vi "Dialog_Arrow Key Handler.vi"(9 "Done Ref":refnum<vi>, 10 "Filter String Ref":refnum<vi>, 11 "Tree Ref":refnum<vi>[](array[refnum])) -> ()   [LabVIEW 2023]
doc: "Called asynchronously, this VI sets the default string (default=\"Filter...\") and the secondary color to the control's text color (default = gray), then monitors the control for a change in focus. When control gains focus, it removes the default string and sets the text to the main text color. When it loses focus, and if string is empty, it sets the value to the default and sets secondary text color.\n\nMake key focus will place the cursor before the default text and handle removing default text if user types any ascii character"
panel:
  in  "Tree":string[](tree)
  in  "Filter String":string
  # "Debug controls:"
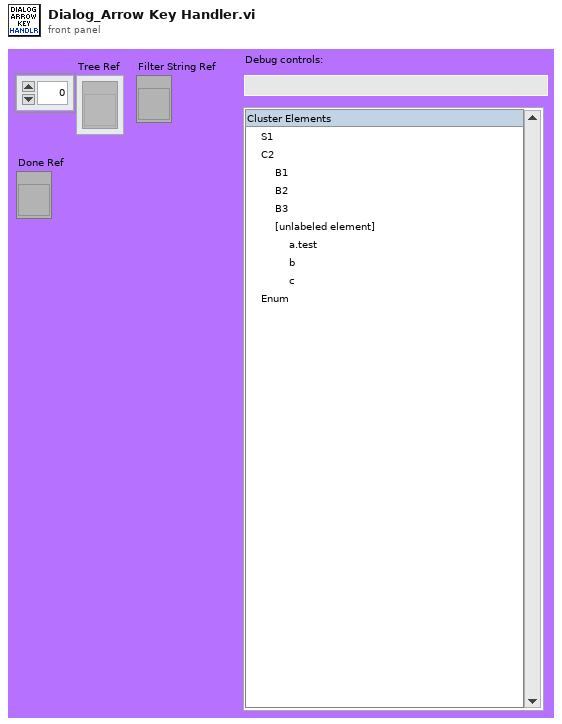
[diagram p1: front panel]
types:
  T1 = typedef "eventvkey.ctl" = enum16{"ASCII", "Enter", "Return", "Shift", "Ctrl", "Alt", "Cmd", "Opt", "Caps", "NumLock", "Clear", "Break", "Up", "Down", "Left", "Right", "Insert", "Delete", "Home", "End", "PageUp", "PageDown", "Escape", "Help", "Pause", "ScrollLock", "F1", "F2", "F3", "F4", "F5", "F6", "F7", "F8", "F9", "F10", "F11", "F12", "F13", "F14", "F15", "F16", "F17", "F18", "F19", "F20", "F21", "F22", "F23", "F24", "Play", "VolumeUp", "VolumeDown", "Mute", "Two Byte Char"}
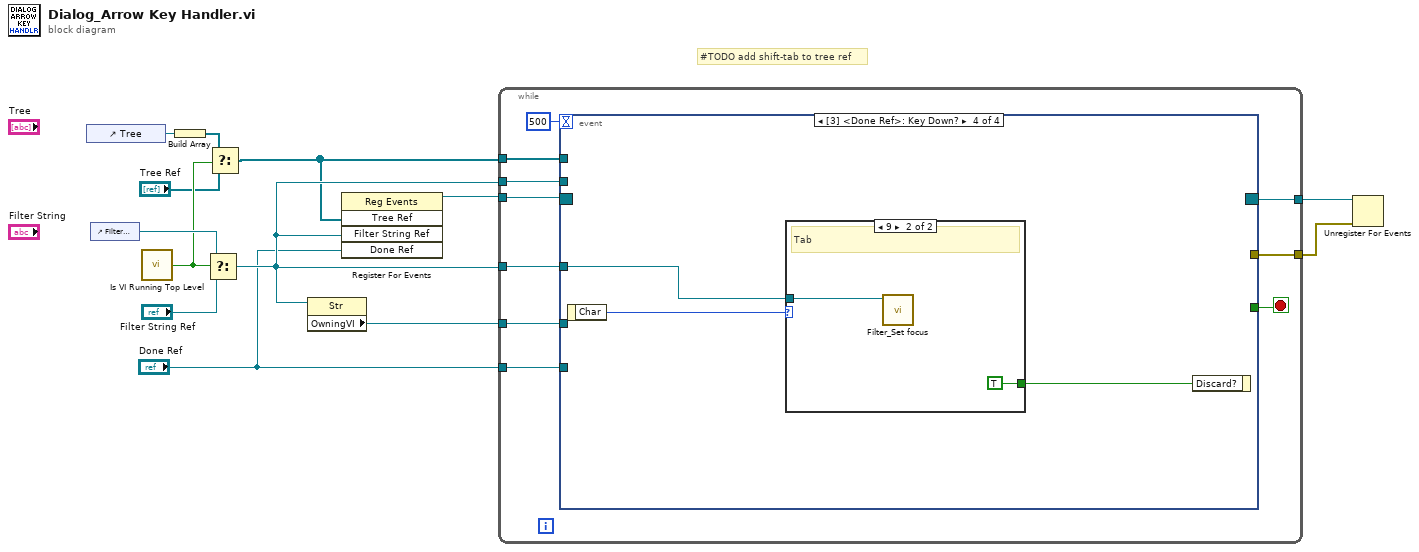
[diagram p0: block diagram]
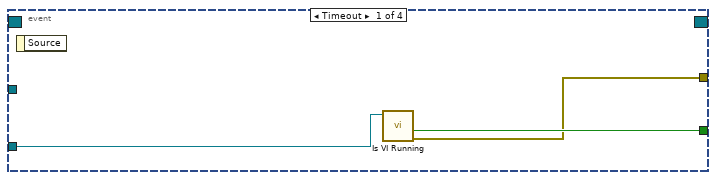
[diagram p2: hidden frame]
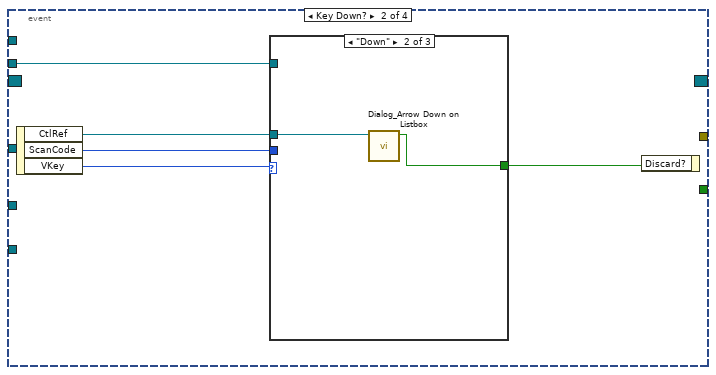
[diagram p3: hidden frame]
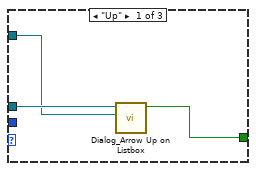
[diagram p4: hidden frame]
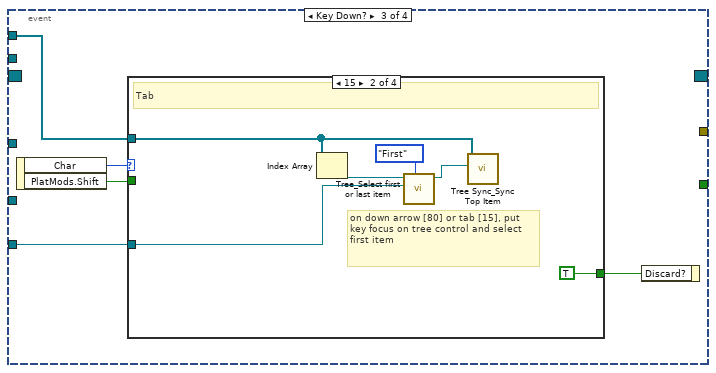
[diagram p6: hidden frame]
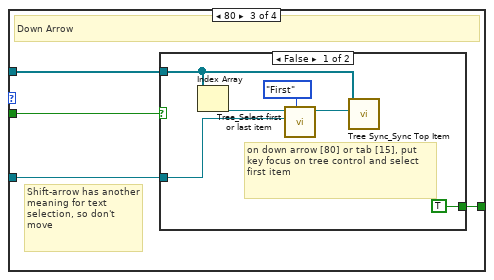
[diagram p8: hidden frame]
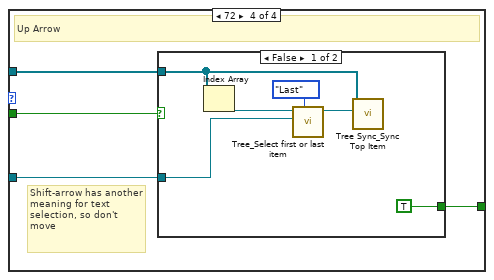
[diagram p10: hidden frame]
diagram:
  # "#TODO add shift-tab to tree ref"
  n1 = control-ref of="Tree"() -> (w9:refnum<vi>)
  n2 = control-ref of="Filter String"() -> (w13:refnum<vi>)
  n3 = call "Is VI Running Top Level.vi"() -> ("Top Level?"=w11:bool)  [unwired: 5 in]
  n4 = Build Array(w9) -> (w2:refnum<vi>[])
  n5 = Select(t=w13, s=w11, f="Filter String Ref") -> (s? t:f=w5:refnum<vi>)
  n6 = Select(t=w2, s=w11, f="Tree Ref") -> (s? t:f=w3:refnum<vi>[])
  n7 = property class="Str"(reference=w5) -> ("OwningVI"=w4:refnum<vi>)  [unwired: 1 in, 2 out]
  n8 = register-events(w3, w5, "Done Ref") -> (reference out=w8:refnum<event-registration>)  [unwired: 2 in, 1 out]
  n9 = while {
    tunnel: w8 -> [w21]
    tunnel: [w20] -> w6
    tunnel: w5 -> [w19]
    tunnel: [w18] -> w7
    tunnel: w5 -> [w17]
    tunnel: w4 -> [w16]
    tunnel: w3 -> [w15]
    tunnel: "Done Ref" -> [w14]
    stop <- w23 stop-if-true
    n10 = event shown="[3] <Done Ref>: Key Down?" {
      selector: w21 -> [_ _ _ _]
      dyn-events: [_ _ _ _] -> w18
      timeout: 500 -> [_ _ _ _]
      tunnel: [w26 _ _ _] -> w23
      tunnel: [w25 _ _ _] -> w20
      tunnel: w19 -> [_ _ _ w69]
      tunnel: w17 -> [_ w27 _ _]
      tunnel: w16 -> [w24 _ _ _]
      tunnel: w15 -> [_ _ w41 _]
      tunnel: w14 -> [_ _ w39 _]
      event Timeout {
        n11 = event-data() -> ()  [unwired: 1 in, 1 out]
        n12 = call "Is VI Running.vi"("VI in"=w24) -> ("error out"=w25:errorcluster, "VI Not Running"=w26:bool)  [unwired: 7 in, 2 out]
      }
      event Key Down? {
        n13 = event-data() -> ("CtlRef"=w29:refnum<vi>, "ScanCode"=w31:i16, "VKey"=w30:T1)  [unwired: 1 in]
        n14 = case shown="\"Down\"" w30 {
          tunnel: w31 -> [_ _ _]
          tunnel: w29 -> [w34 w36 _]
          tunnel: [w32 w35 _] -> w28
          tunnel: w27 -> [w33 _ _]
          frame "Up" {
            n15 = call "Dialog_Arrow Up on Listbox.vi"("String Ref"=w33, "TreeControl in"=w34) -> ("discard"=w32:bool)  [unwired: 9 in]
          }
          frame "Down" {
            n16 = call "Dialog_Arrow Down on Listbox.vi"("TreeControl in"=w36) -> ("discard"=w35:bool)  [unwired: 10 in]
          }
          frame Default {
          }
        }
        n17 = event-data("Discard?"=w28) -> ()  [unwired: 1 in, 1 out]
      }
      event Key Down? {
        n18 = event-data() -> ("Char"=w40:i16, "PlatMods.Shift"=w38:bool)  [unwired: 1 in]
        n19 = case shown="15" w40 {
          tunnel: w41 -> [_ w47 w51 w61]
          tunnel: w38 -> [_ _ w50 w60]
          tunnel: w39 -> [_ w43 w49 w59]
          tunnel: [_ TRUE ("Discard?") w48 w58] -> w37
          frame Default {
          }
          frame 15 {
            # "on down arrow [80] or tab [15], put key focus on tree control and select first item"
            # "Tab"
            n20 = Index Array(array=w47) -> (element=w44:refnum<vi>)  [unwired: 1 in]
            n21 = call "Tree_Select first or last item.vi"("Select Item"=enum16{"First", "Last"}."First", "Done Ref"=w43, "Tree Ref"=w44) -> ("Tree Ref Out"=w45:refnum<vi>)  [unwired: 7 in, 1 out]
            n22 = call "Tree Sync_Sync Top Item.vi"("Changed Tree Control Ref"=w45, "All Tree Control Refs"=w47) -> ()  [unwired: 9 in, 1 out]
          }
          frame 80 {
            # "Shift-arrow has another meaning for text selection, so don't move"
            # "Down Arrow"
            n23 = case shown="False" w50 {
              tunnel: w51 -> [w55 _]
              tunnel: w49 -> [w53 _]
              tunnel: [TRUE ("Discard?") _] -> w48
              frame False {
                # "on down arrow [80] or tab [15], put key focus on tree control and select first item"
                n24 = Index Array(array=w55) -> (element=w54:refnum<vi>)  [unwired: 1 in]
                n25 = call "Tree_Select first or last item.vi"("Select Item"=enum16{"First", "Last"}."First", "Done Ref"=w53, "Tree Ref"=w54) -> ("Tree Ref Out"=w56:refnum<vi>)  [unwired: 7 in, 1 out]
                n26 = call "Tree Sync_Sync Top Item.vi"("Changed Tree Control Ref"=w56, "All Tree Control Refs"=w55) -> ()  [unwired: 9 in, 1 out]
              }
              frame True {
              }
            }
          }
          frame 72 {
            # "Shift-arrow has another meaning for text selection, so don't move"
            # "Up Arrow"
            n27 = case shown="False" w60 {
              tunnel: w61 -> [w65 _]
              tunnel: w59 -> [w63 _]
              tunnel: [TRUE ("Discard?") _] -> w58
              frame False {
                n28 = Index Array(array=w65) -> (element=w64:refnum<vi>)  [unwired: 1 in]
                n29 = call "Tree_Select first or last item.vi"("Select Item"=enum16{"First", "Last"}."Last", "Done Ref"=w63, "Tree Ref"=w64) -> ("Tree Ref Out"=w66:refnum<vi>)  [unwired: 7 in, 1 out]
                n30 = call "Tree Sync_Sync Top Item.vi"("Changed Tree Control Ref"=w66, "All Tree Control Refs"=w65) -> ()  [unwired: 9 in, 1 out]
              }
              frame True {
              }
            }
          }
        }
        n31 = event-data("Discard?"=w37) -> ()  [unwired: 1 in, 1 out]
      }
      event Key Down? {
        n32 = event-data() -> ("Char"=w70:i16)  [unwired: 1 in]
        n33 = case shown="9" w70 {
          tunnel: [_ TRUE ("Discard?")] -> w68
          tunnel: w69 -> [_ w71]
          frame 0, Default {
          }
          frame 9 {
            # "Tab"
            n34 = call "Filter_Set focus.vi"("Fillter String Ref"=w71) -> ()  [unwired: 10 in, 1 out]
          }
        }
        n35 = event-data("Discard?"=w68) -> ()  [unwired: 1 in, 1 out]
      }
    }
  }
  n36 = Unregister For Events(event registration refnum=w7, error in=w6) -> ()  [unwired: 1 out]
